vi "Outputs SW Set.vi"(7 "Auto CMD":T1 {"Target Auto Angle" scale format="%.3f"; "Direction"."Rotate(Yaw) CCW 1 CW -1" scale=1.0..-1.0; "Direction"."Traverse"."Angle" scale format="%.3f"; "Direction"."Traverse"."Velocity" scale=-1.0..1.0 scale format="%.1f"}, 8 "Current Time":timestamp format="%<%x %.3X>T", 9 "System Config":T8={"System Ver"=0, "Auto Angle PID"={"Gains"={"P"=0.1, "I"=0.0, "D"=0.0, "F"=0.0}, "Error Allowed"={"High"=0.0, "Low"=0.0}, "I Zone"={"High"=0.0, "Low"=0.0}, "Peak Out 0-1"={"High"=0.0, "Low"=0.0}, "Max I Accu"={"High"=0.0, "Low"=0.0}}, "Frame"={"Length"=33.0, "Width"=18.0}, "Drive Data"={"CPR"=14.0, "RevMotor/Wheel"=6.67, "Wheel Diameter (in)"=4.0}, "Speed Full Scale"=5000.0, "Steer Data"={"CPR"=1024.0}} {"Auto Angle PID"."Max I Accu"."Low" format="%#.8f"; "Auto Angle PID"."Max I Accu"."High" format="%#.8f"; "Auto Angle PID"."Gains"."F" format="%#.8f"; "Auto Angle PID"."Gains"."D" format="%#.8f"; "Auto Angle PID"."Gains"."I" format="%#.8f"; "Auto Angle PID"."Gains"."P" format="%#.8f"; "Auto Angle PID"."Error Allowed"."Low" format="%#.8f"; "Auto Angle PID"."Error Allowed"."High" format="%#.8f"; "Auto Angle PID"."I Zone"."Low" format="%#.8f"; "Auto Angle PID"."I Zone"."High" format="%#.8f"; "Auto Angle PID"."Peak Out 0-1"."Low" format="%#.8f"; "Auto Angle PID"."Peak Out 0-1"."High" format="%#.8f"}, 10 "Sensor Values":T16 {"Swerve Read"."Back Right"."Angle" scale format="%.3f"; "Swerve Read"."Back Right"."Velocity" scale=-1.0..1.0 scale format="%.1f"; "Swerve Read"."Back Left"."Angle" scale format="%.3f"; "Swerve Read"."Back Left"."Velocity" scale=-1.0..1.0 scale format="%.1f"; "Swerve Read"."Front Left"."Angle" scale format="%.3f"; "Swerve Read"."Front Left"."Velocity" scale=-1.0..1.0 scale format="%.1f"; "Swerve Read"."Front Right"."Angle" scale format="%.3f"; "Swerve Read"."Front Right"."Velocity" scale=-1.0..1.0 scale format="%.1f"; "Pigeon Heading" scale format="%.3f"}, 11 "SW Output":T15) -> (3 "SW Output Out":T15, 5 "Auto CMD Out":T1 {"Target Auto Angle" scale format="%.3f"; "Direction"."Rotate(Yaw) CCW 1 CW -1" scale=1.0..-1.0; "Direction"."Traverse"."Angle" scale format="%.3f"; "Direction"."Traverse"."Velocity" scale=-1.0..1.0 scale format="%.1f"})   [LabVIEW 2023, in "Swerve AM_ACT.lvlib"]
uses:
  Swerve AM_ACT.lvlib
  Cluster_HW Output Values.ctl
  Shared Code/TypeDefs/Dial_Compase heading unit circle CCW positive.ctl
  Shared Code/TypeDefs/Cluster_Swerve 4 Steer and Velocity.ctl
  Shared Code/TypeDefs/Cluster_Module Velocity-Direction-Rotations.ctl
  Shared Code/TypeDefs/Level_Velocity plus-minus 1.ctl
  Cluster_System Output Data.ctl
  Cluster_System Config_Values.ctl
  Shared Code/TypeDefs/Cluster_SW PID Config.ctl
  Shared Code/TypeDefs/Cluster_PID Gains.ctl
  Shared Code/TypeDefs/Cluster_High-Low.ctl
  Type Defs/Cluster_Length and Width.ctl
  Shared Code/TypeDefs/Cluster_Config_Swerve_Drive Param.ctl
  Shared Code/TypeDefs/Cluster_Config_Swerve_Steer Parm.ctl
  Cluster_CMD_ACT_Data.ctl
  ENUM_CMD_Mode Select.ctl
  Shared Code/TypeDefs/Cluster_CMD_Direction Data.ctl
  Shared Code/TypeDefs/Cluster_X-Y.ctl
  b2c39663-cabd-45a6-97f7-b6bfb450ad48.vi
panel:
  # "\"Front\" of Robot"
  # "Index 1"
  # "Index 0"
  # "Index 3"
  # "Index 2"
  # "Right Hand Rule"
  # "X"
  # "+CCW"
  # "Y"
  # "(0,0)"
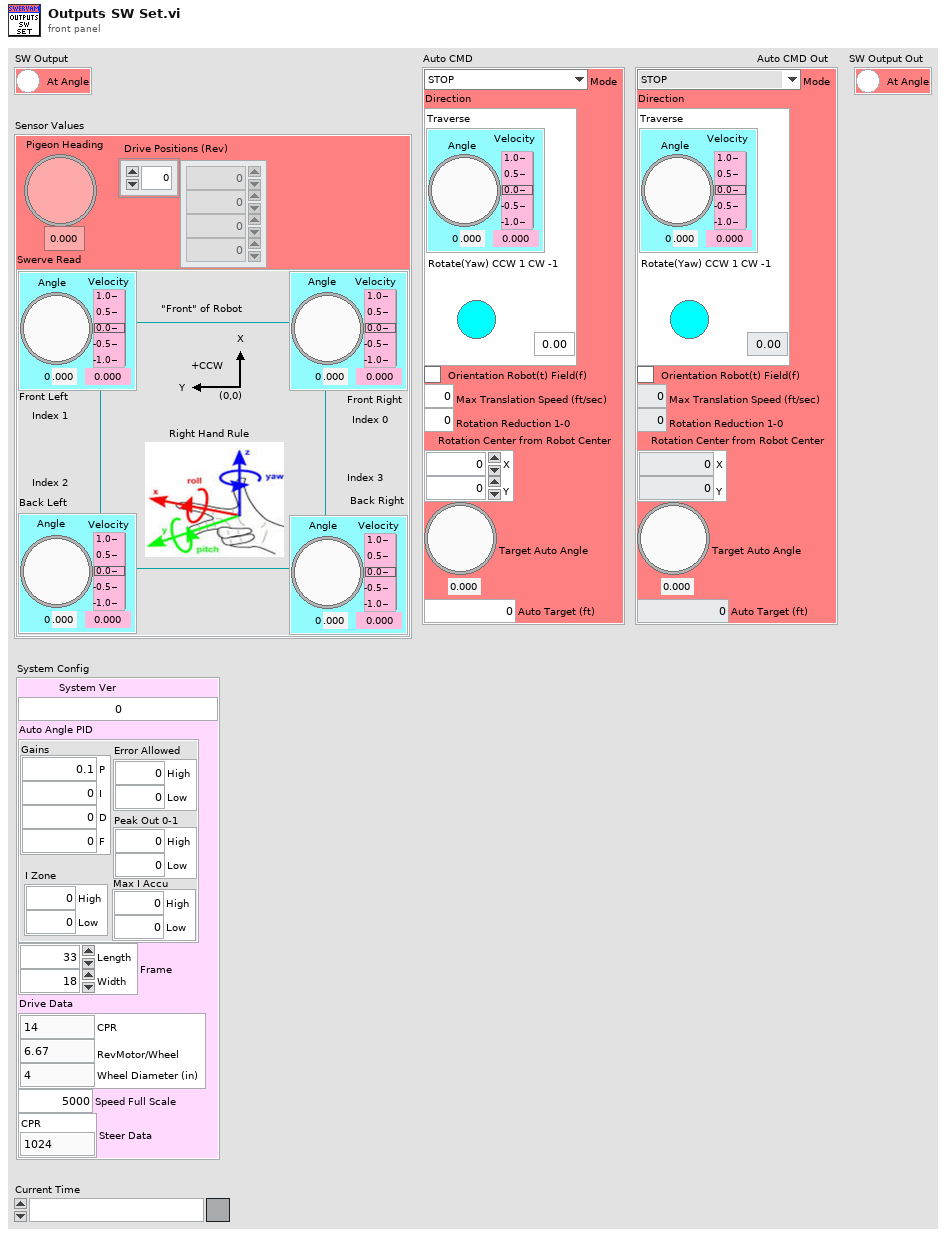
[diagram p1: front panel]
types:
  T1 = typedef "Swerve AM_ACT.lvlib/Cluster_CMD_ACT_Data.ctl" = cluster{"Mode":T2, "Direction":T3, "Orientation Robot(t) Field(f)":bool, "Max Translation Speed (ft/sec)":dbl, "Rotation Reduction 1-0":dbl, "Rotation Center from Robot Center":T7, "Target Auto Angle":T6, "Auto Target (ft)":dbl}
  T2 = typedef "Swerve AM_ACT.lvlib/ENUM_CMD_Mode Select.ctl" = enum16{"STOP", "Move", "Turret Manual", "Trans Manual Angle Auto", "Turret Auto Angle"}
  T3 = typedef "Cluster_CMD_Direction Data.ctl" = cluster{"Traverse":T4, "Rotate(Yaw) CCW 1 CW -1":dbl}
  T4 = typedef "Cluster_Module Velocity-Direction-Rotations.ctl" = cluster{"Velocity":T5, "Angle":T6, "Rotations Count":dbl}
  T5 = typedef "Level_Velocity plus-minus 1.ctl" = dbl
  T6 = typedef "Dial_Compase heading unit circle CCW positive.ctl" = dbl
  T7 = typedef "Cluster_X-Y.ctl" = cluster{"X":dbl, "Y":dbl}
  T8 = typedef "Swerve AM_ACT.lvlib/Cluster_System Config_Values.ctl" = cluster{"System Ver":u64, "Auto Angle PID":T9, "Frame":T12, "Drive Data":T13, "Speed Full Scale":dbl, "Steer Data":T14}
  T9 = typedef "Cluster_SW PID Config.ctl" = cluster{"Gains":T10, "Error Allowed":T11, "I Zone":T11, "Peak Out 0-1":T11, "Max I Accu":T11}
  T10 = typedef "Cluster_PID Gains.ctl" = cluster{"P":dbl, "I":dbl, "D":dbl, "F":dbl}
  T11 = typedef "Cluster_High-Low.ctl" = cluster{"High":dbl, "Low":dbl}
  T12 = typedef "Cluster_Length and Width.ctl" = cluster{"Length":dbl, "Width":dbl}
  T13 = typedef "Cluster_Config_Swerve_Drive Param.ctl" = cluster{"CPR":dbl, "RevMotor/Wheel":dbl, "Wheel Diameter (in)":dbl}
  T14 = typedef "Cluster_Config_Swerve_Steer Parm.ctl" = cluster{"CPR":dbl}
  T15 = typedef "Swerve AM_ACT.lvlib/Cluster_System Output Data.ctl" = cluster{"At Angle":bool}
  T16 = typedef "Swerve AM_ACT.lvlib/Cluster_HW Output Values.ctl" = cluster{"Pigeon Heading":T6, "Swerve Read":T17, "Drive Positions (Rev)":dbl[]}
  T17 = typedef "Cluster_Swerve 4 Steer and Velocity.ctl" = cluster{"Front Right":T4, "Front Left":T4, "Back Left":T4, "Back Right":T4}
  T18 = typedef "NUM_Rotate Input.ctl" = dbl
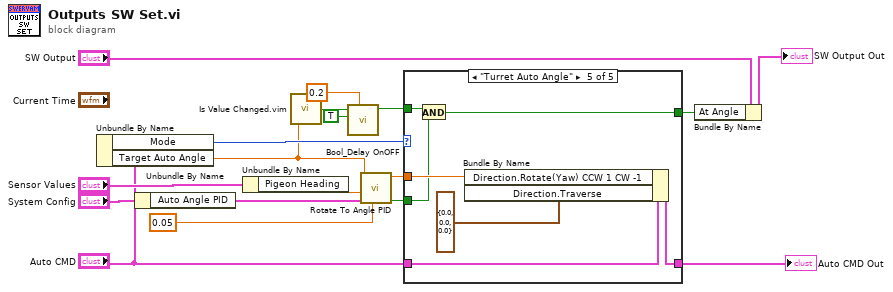
[diagram p0: block diagram]
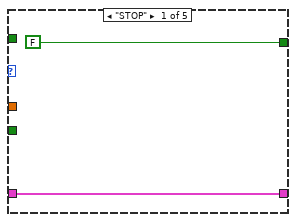
[diagram p2: hidden frame]
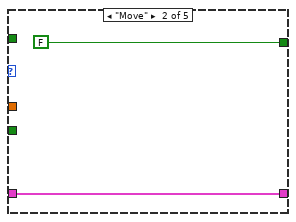
[diagram p3: hidden frame]
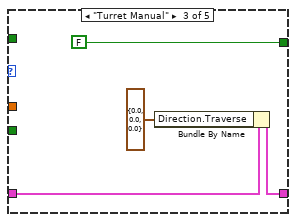
[diagram p4: hidden frame]
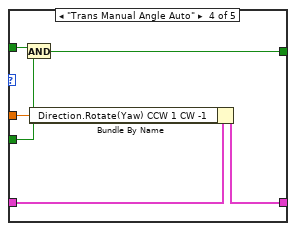
[diagram p5: hidden frame]
diagram:
  n1 = Unbundle By Name("Auto CMD") -> ("Mode"=w7:T2, "Target Auto Angle"=w6:T6)
  n2 = Unbundle By Name("System Config") -> ("Auto Angle PID"=w12:T9)
  n3 = Unbundle By Name("Sensor Values") -> ("Pigeon Heading"=w14:T6)
  n4 = call "Is Value Changed.vim"("value"=w6) -> ("changed or first call?"=w5:bool)
  n5 = call "Bool_Delay OnOFF.vi"("Delay Time(S)"=0.2, "Delay On(t) Off(f)"=TRUE, "Input"=w5) -> ("Output"=w1:bool)  [unwired: 7 in, 1 out]
  n6 = call "Rotate To Angle PID.vi"("Target Cycle Time(S)"=0.05, "PID Config"=w12, "Current Yaw"=w14, "Target Yaw"=w6) -> ("At Angle Out"=w2:bool, "Direction.Rotate(Yaw) CCW 1 CW -1 Out"=w9:T18)  [unwired: 5 in, 1 out]
  n7 = case shown="\"Turret Auto Angle\"" w7 {
    tunnel: [FALSE ("Out Data 1") FALSE ("Out Data 1") FALSE ("Out Data 1") w27 w34] -> w16
    tunnel: "Auto CMD" -> [w19 w21 w24 w31 w38]
    tunnel: [w19 w21 w25 w32 w39] -> w10
    tunnel: w9 -> [_ _ _ w30 w37]
    tunnel: w2 -> [_ _ _ w28 w35]
    tunnel: w1 -> [_ _ _ w29 w36]
    frame "STOP" {
    }
    frame "Move" {
    }
    frame "Turret Manual" {
      n8 = Bundle By Name(cluster=w24, "Direction.Traverse"=T4 {"Velocity"=0.0, "Angle"=0.0, "Rotations Count"=0.0}) -> (w25:T1)
    }
    frame "Trans Manual Angle Auto" {
      n9 = And(x=w29, y=w28) -> (x .and. y?=w27:bool)
      n10 = Bundle By Name(cluster=w31, "Direction.Rotate(Yaw) CCW 1 CW -1"=w30) -> (w32:T1)
    }
    frame "Turret Auto Angle" {
      n11 = And(x=w36, y=w35) -> (x .and. y?=w34:bool)
      n12 = Bundle By Name(cluster=w38, "Direction.Rotate(Yaw) CCW 1 CW -1"=w37, "Direction.Traverse"=T4 {"Velocity"=0.0, "Angle"=0.0, "Rotations Count"=0.0}) -> (w39:T1)
    }
  }
  "Auto CMD Out" <- w10
  n13 = Bundle By Name(cluster="SW Output", "At Angle"=w16) -> (→"SW Output Out":T15)
